vi "44_All_Area.vi"() -> ()   [LabVIEW 2018]
panel:
  in  "Stop":bool caption="Stop (F)"
  out "Image Out":T1(plugin-control)
  # "選出所有目標"
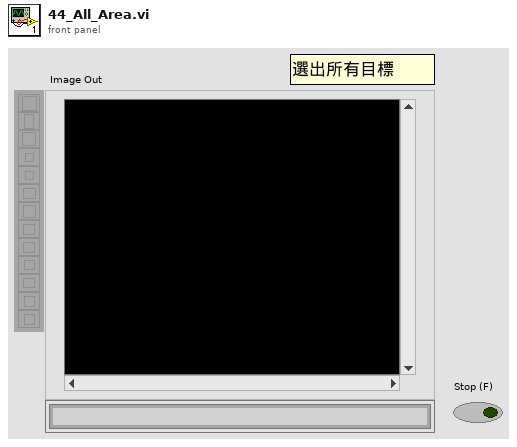
[diagram p1: front panel]
types:
  T1 = typedef "IMAQ Image.ctl" = refnum<image>
  T2 = cluster{"Left":dbl, "Top":dbl, "Right":dbl, "Bottom":dbl}
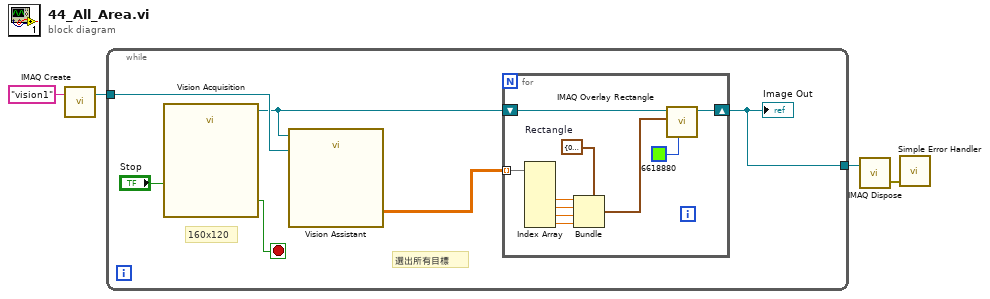
[diagram p0: block diagram]
diagram:
  n1 = call "IMAQ Create"("Image Name"="vision1") -> ("New Image"=w3:T1)  [unwired: 4 in, 1 out]
  n2 = while {
    tunnel: w3 -> [w8]
    tunnel: [w5] -> w1
    stop <- w9 stop-if-true
    # "選出所有目標"
    # "160x120"
    n3 = call "Vision Acquisition"("Stop (F)"="Stop") -> ("Image Out"=w7:T1, "Stopped"=w9:bool)  [unwired: 24 in, 1 out]
    n4 = call "Vision Assistant"("Image In"=w7, "Image Dst"=w8) -> ("Particle Measurements (Pixels) (Particle Analysis 1)"=w6:dbl[][])  [unwired: 22 in, 3 out]
    n5 = for {
      tunnel: w6 -> [w13] mode=indexing
      shift-right: [w11] -> w5
      shift-left: w7 -> [w12]
      w14 = T2 {"Left"=0.0, "Top"=0.0, "Right"=0.0, "Bottom"=0.0}  # Rectangle
      n6 = Index Array "Index Array"(array=w13) -> (element #3=w15:dbl, element #4=w16:dbl, element #5=w17:dbl, element #6=w18:dbl)  [unwired: 6 in, 2 out]
      n7 = Bundle "Bundle"(cluster=w14, "Left"=w15, "Top"=w16, "Right"=w17, "Bottom"=w18) -> (w19:T2)
      n8 = call "IMAQ Overlay Rectangle"("Color"=u32 6618880, "Rectangle"=w19, "Image"=w12) -> ("Image Out"=w11:T1)  [unwired: 7 in, 1 out]
    }
    "Image Out" <- w5
  }
  n9 = call "IMAQ Dispose"("Image"=w1) -> ("error out"=w2:errorcluster)  [unwired: 5 in]
  n10 = call <vilib>:"Simple Error Handler.vi"("error in (no error)"=w2) -> ()  [unwired: 4 in, 5 out]
